vi "Get Next Step.vi"(8 "error in (no error)":errorcluster, 9 "Status Text In":string, 10 "Current Step in":i32, 11 "Sequence In":T2[](array[typedef])) -> (0 "error out":errorcluster, 1 "Status Text Out":string, 2 "Current Step out":i32, 3 "Sequence Out":T2[](array[typedef]), 5 "Enum":T1)   [LabVIEW 2018]
doc: "This VI determines whether the sequence is complete or whether there are more steps to execute. When done, it returns the next state of the Sequence Engine."
uses:
  Message Queue/Message Cluster (string).ctl
  Message Queue/Message (enum).ctl
  controls/Sequence Engine State.ctl
  Message Queue/Message Queue.lvlib
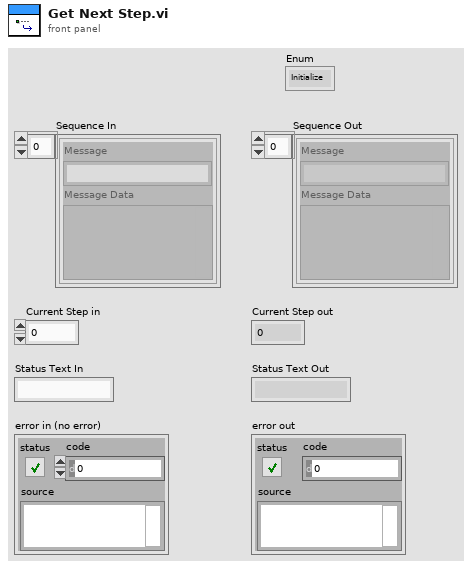
[diagram p1: front panel]
types:
  T1 = typedef "Message Queue.lvlib/Message (enum).ctl" = enum16{"Initialize", "Idle", "Running", "Stop", "Pause", "Resume", "Load Sequence File", "Load Sequence from UI", "Save Sequence File"}
  T2 = typedef "Message Queue.lvlib/Message Cluster (string).ctl" = cluster{"Message":string, "Message Data":variant}
  T3 = typedef "Sequence Engine State.ctl" = enum16{"Idle", "Running", "Stop", "Pause", "Resume", "Load Sequence"}
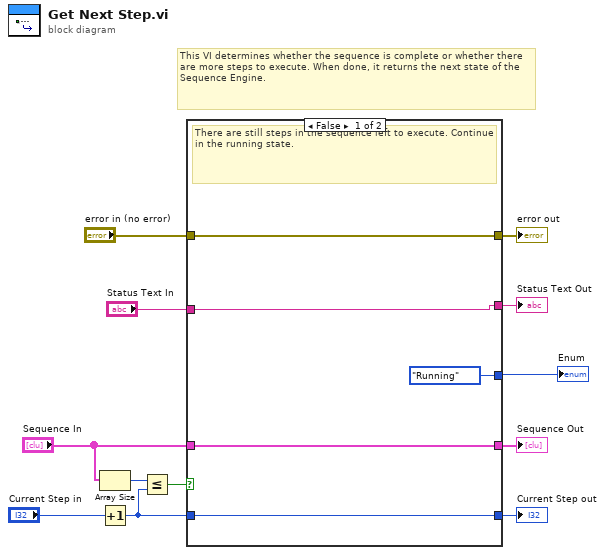
[diagram p0: block diagram]
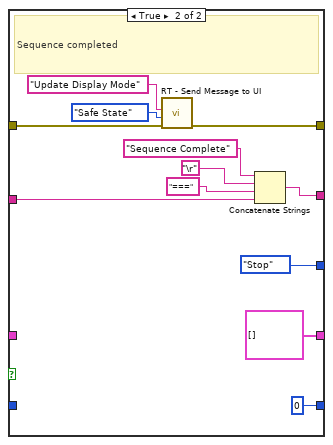
[diagram p2: hidden frame]
diagram:
  # "This VI determines whether the sequence is complete or whether there are more steps to execute. When done, it returns the next state of the Sequence Engine."
  n1 = Array Size(array="Sequence In") -> (size(s)=w3:i32)
  n2 = Increment(x="Current Step in") -> (x+1=w5:i32)
  n3 = Less Or Equal?(x=w3, y=w5) -> (x <= y?=w4:bool)
  n4 = case shown="False" w4 {
    tunnel: w5 -> [w16 _]
    tunnel: "Sequence In" -> [w17 _]
    tunnel: [w17 T2[] []] -> w7
    tunnel: [w16 0 ("Current Step")] -> w8
    tunnel: [Sequence_Engine_State."Running" ("Sequence Engine State") Message_(enum)."Stop" ("Enum")] -> w1
    tunnel: "Status Text In" -> [w14 w26]
    tunnel: [w14 w27] -> w10
    tunnel: "error in (no error)" -> [w13 w25]
    tunnel: [w13 w24] -> w12
    frame False {
      # "There are still steps in the sequence left to execute. Continue in the running state."
    }
    frame True {
      # "Sequence completed"
      n5 = call "RT - Send Message to UI.vi"("error in (no error)"=w25, "Message Data"=enum16{"Safe State", "Control (PID)"}."Safe State" ("New State"), "Message"="Update Display Mode") -> ("error out"=w24:errorcluster)  [unwired: 8 in]
      n6 = Concatenate Strings("Sequence Complete" ("string"), "\r", "===" ("string"), w26) -> (w27:string)
    }
  }
  "error out" <- w12
  "Status Text Out" <- w10
  "Current Step out" <- w8
  "Sequence Out" <- w7
  "Enum" <- w1
